vi "Save Background.vi"(8 "error in":errorcluster, 10 "File Path":path, 11 "BigMAQ in":refnum<class "BigMAQ.lvclass">) -> (0 "error out":errorcluster, 3 "BigMAQ out":refnum<class "BigMAQ.lvclass">)   [LabVIEW 2019, in "BigMAQ.lvclass"]
uses:
  BigMAQ.lvclass
  BigMAQ.lvclass/BigMAQ.ctl
  <userlib>/_OpenG.lib/md5/md5.llb/MD5 Message Digest (Binary String)__ogtk.vi
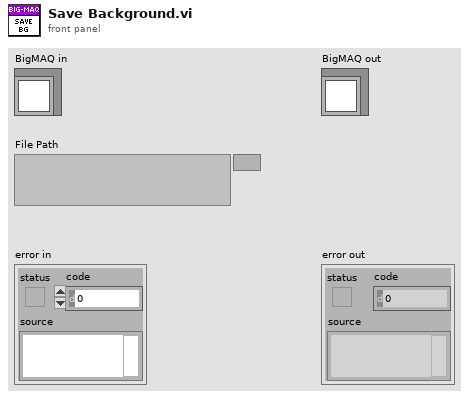
[diagram p1: front panel]
types:
  T1 = typedef "Image Type" = u32
  T2 = typedef "IMAQ Image.ctl" = refnum<image>
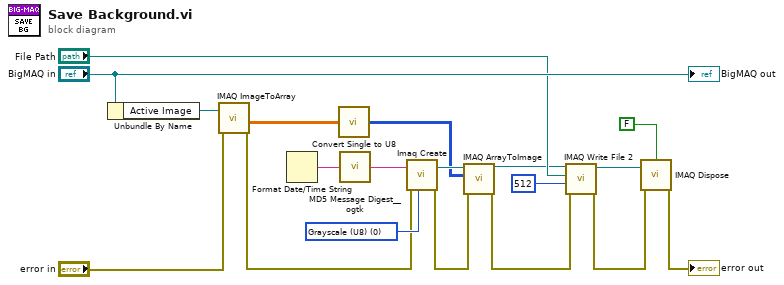
[diagram p0: block diagram]
diagram:
  w12 = T1 0 items=["Grayscale (U8)", "Grayscale (I16)", "Grayscale (SGL)", "Complex (CSG)", "RGB (U32)", "HSL (U32)", "RGB (U64)", "Grayscale (U16)"] ("Image Type")
  n1 = Unbundle By Name("BigMAQ in") -> ("Active Image"=w9:T2)
  n2 = call "IMAQ ImageToArray"("error in (no error)"="error in", "Image"=w9) -> ("Image Pixels (Float)"=w2:sgl[][], "error out"=w5:errorcluster)  [unwired: 2 in, 3 out]
  n3 = Format Date/Time String() -> (date/time string=w18:string)  [unwired: 3 in]
  n4 = call "Convert Single to U8.vi"("Image Pixels (Float)"=w2) -> ("Image Pixels (U8)"=w1:u8[][])
  n5 = call-poly <userlib>:"MD5 Message Digest__ogtk.vi"("Message"=w18) -> ("MD5 Message Digest"=w7:string)
  n6 = call "Imaq Create"("Image Name"=w7, "Image Type"=w12, "error in (no error)"=w5) -> ("New Image"=w8:T2, "error out"=w4:errorcluster)  [unwired: 2 in]
  n7 = call "IMAQ ArrayToImage"("error in (no error)"=w4, "Image Pixels (U8)"=w1, "Image"=w8) -> ("error out"=w3:errorcluster, "Image Out"=w11:T2)  [unwired: 7 in]
  n8 = call-poly "IMAQ Write File 2"("error in (no error)"=w3, "Image Quality"=u32 512, "File Path"="File Path", "Image"=w11) -> ("error out"=w10:errorcluster, "Image Out (duplicate)"=w16:T2)  [unwired: 6 in]
  n9 = call "IMAQ Dispose"("All Images? (No)"=FALSE, "Image"=w16, "error in (no error)"=w10) -> ("error out"=→"error out":errorcluster)  [unwired: 3 in]
  "BigMAQ out" <- "BigMAQ in"
